vi "Get DSF File Version.vi"() -> (3 "dsf":T1)   [LabVIEW 2017, in "Data Sharing Framework Configuration.lvlib"]
uses:
  Data Sharing Framework Configuration.lvlib
  Public/Controls/DSF Version Info.ctl
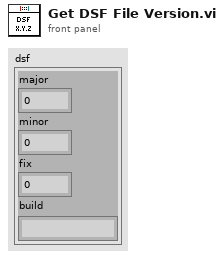
[diagram p1: front panel]
types:
  T1 = typedef "Data Sharing Framework Configuration.lvlib/DSF Version Info.ctl" = cluster{"major":u32, "minor":u32, "fix":u32, "build":string}
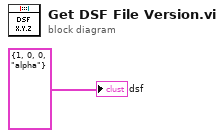
[diagram p0: block diagram]
diagram:
  "dsf" <- T1 {"major"=1, "minor"=0, "fix"=0, "build"="alpha"} ("dsf")
